vi "Flatten.vi"(8 "error in":errorcluster, 10 "Cluster":variant, 11 "JSON in":refnum<class "JSON.lvclass">) -> (0 "error out":errorcluster, 2 "JSON String":string, 3 "JSON out":refnum<class "JSON.lvclass">)   [LabVIEW 2017, in "Reports.lvlib" / "JSON.lvclass"]
doc: "This method serves for flatten\ndata to JSON string"
uses:
  JSON.lvclass
  <vilib>/addons/_JKI.lib/Serialization/JSON/JKI JSON Serialization.lvlib
  <vilib>/addons/_JKI.lib/Serialization/JSON/Library/Timestamp Options.ctl
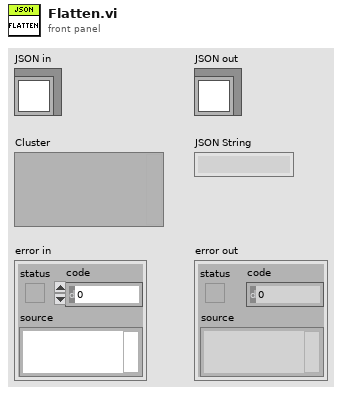
[diagram p1: front panel]
types:
  T1 = typedef "JKI JSON Serialization.lvlib/Timestamp Options.ctl" = cluster{"Convert Timestamps":bool, "UTC":bool}
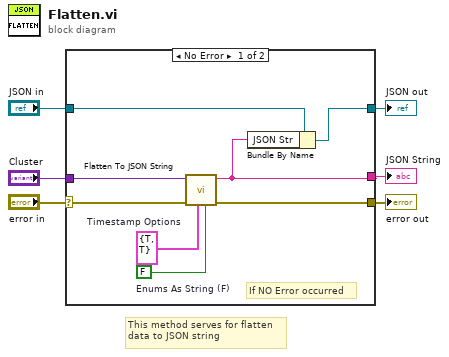
[diagram p0: block diagram]
diagram:
  # "This method serves for flatten\ndata to JSON string"
  n1 = case shown="No Error" "error in" {
    selector: "error in" -> [w13 w16]
    tunnel: [w12 w16] -> w5
    tunnel: [w8 w15] -> w3
    tunnel: "JSON in" -> [w9 w15]
    tunnel: "Cluster" -> [w14 _]
    tunnel: [w7 _] -> w1
    frame No Error {
      w10 = FALSE  # Enums As String (F)
      w11 = T1 {"Convert Timestamps"=TRUE, "UTC"=TRUE}  # Timestamp Options
      # "If NO Error occurred"
      n2 = call <vilib>:"Flatten To JSON String.vi"("Enums As String (F)"=w10, "Timestamp Options"=w11, "error in (no error)"=w13, "Variant"=w14) -> ("error out"=w12:errorcluster, "JSON String"=w7:string)  [unwired: 6 in]
      n3 = Bundle By Name(cluster=w9, "JSON Str"=w7) -> (w8:refnum<class "JSON.lvclass">)
    }
    frame Error {
    }
  }
  "error out" <- w5
  "JSON out" <- w3
  "JSON String" <- w1
